vi "Add Image.vi"(0 "Image Ref":T1, 11 "Error In":errorcluster) -> (15 "Error Out":errorcluster)   [LabVIEW 2020]
uses:
  <vilib>/vision/Image Controls.llb/IMAQ Image.ctl
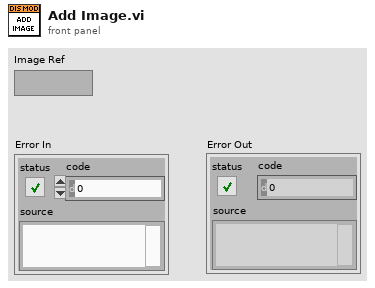
[diagram p1: front panel]
types:
  T1 = typedef "IMAQ Image.ctl" = refnum<image>
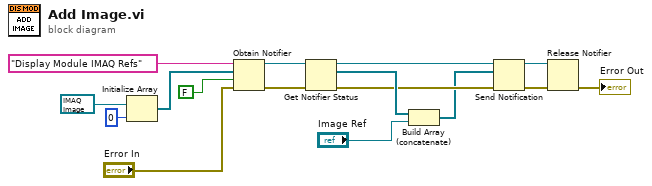
[diagram p0: block diagram]
diagram:
  n1 = Initialize Array(T1 refnum ("New Image"), 0 ("dimension size")) -> (w12:T1[])
  n2 = Obtain Notifier(name (unnamed)="Display Module IMAQ Refs", notification data type=w12, create if not found? (T)=FALSE, error in (no error)="Error In") -> (notifier out=w3:refnum<notifier>, error out=w2:errorcluster)  [unwired: 1 out]
  n3 = Get Notifier Status(notifier=w3, error in (no error)=w2) -> (notifier out=w10:refnum<notifier>, current notification=w11:T1[], error out=w9:errorcluster)  [unwired: 2 out]
  n4 = Build Array (concatenate)(w11, "Image Ref") -> (w8:T1[])
  n5 = Send Notification(notification=w8, notifier=w10, error in (no error)=w9) -> (notifier out=w6:refnum<notifier>, error out=w5:errorcluster)
  n6 = Release Notifier(notifier=w6, error in (no error)=w5) -> (error out=→"Error Out":errorcluster)  [unwired: 1 in, 2 out]
